vi "Export Simplified Image.vi"(11 "Control Ref Queue":T2) -> ()   [LabVIEW 2020, in "XY Plot Matrix.lvclass"]
uses:
  <vilib>/Math Plots/2D Math Plots/XY Plot Matrix/XY Plot Matrix/XY Plot Matrix.lvclass
  <vilib>/Math Plots/2D Math Plots/2D Plot/Action String/XYPlotMatrix Ctrl Act Queue.ctl
  <vilib>/Math Plots/2D Math Plots/2D Plot/Action String/XYPlotMatrix Ctrl Act Cluster.ctl
  <vilib>/Math Plots/2D Math Plots/2D Plot/Action String/2DMathPlot State Class.ctl
panel:
  in  "Warning Message":string="File path is invalid."
  in  "Save":string="Save"
  in  "Export":string="Export"
  in  "Tab Control":enum32{"Appearance", "Input & Output"}(tab)
  in  "To Clipboard":bool=TRUE
  in  "To File":bool
  in  "Help":bool
  in  "Cancel":bool
  in  "OK":bool
  in  "Hide Grid":bool
  in  "Path":path
  in  "File Format":T1(radio)
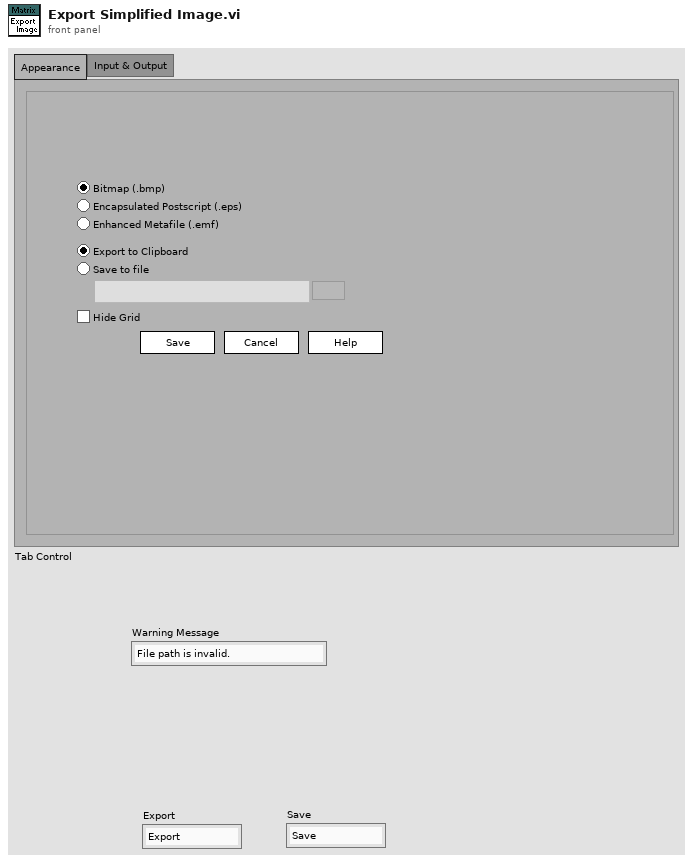
[diagram p1: front panel]
types:
  T1 = enum32{"Bitmap", "Postscript", "Metafile", "Mac PICT (.pict)"}
  T2 = typedef "XYPlotMatrix Ctrl Act Queue.ctl" = refnum<queue>
  T3 = enum8{"Enabled", "Disabled", "Disabled and Grayed Out"}
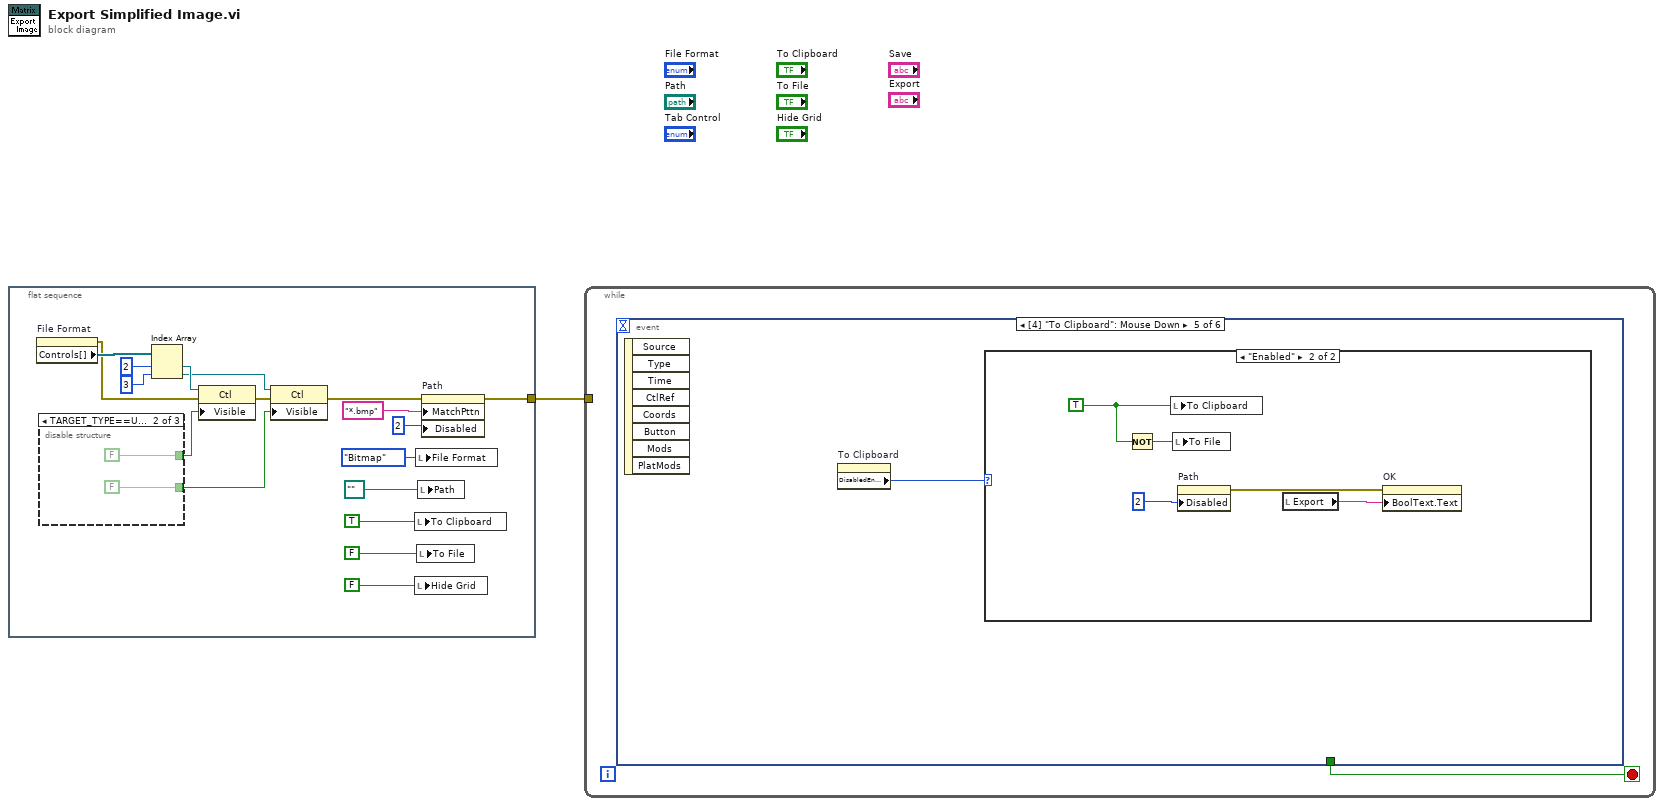
[diagram p0: block diagram]
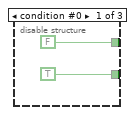
[diagram p2: hidden frame]
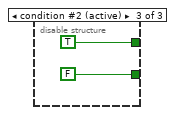
[diagram p3: hidden frame]
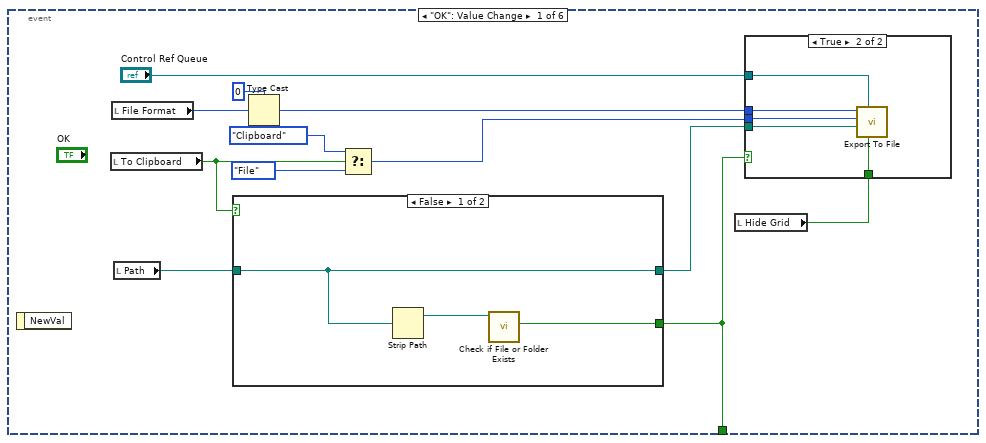
[diagram p4: hidden frame]
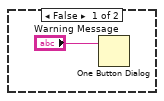
[diagram p5: hidden frame]
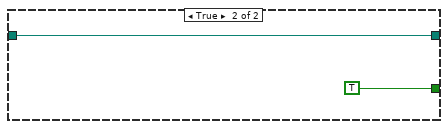
[diagram p6: hidden frame]
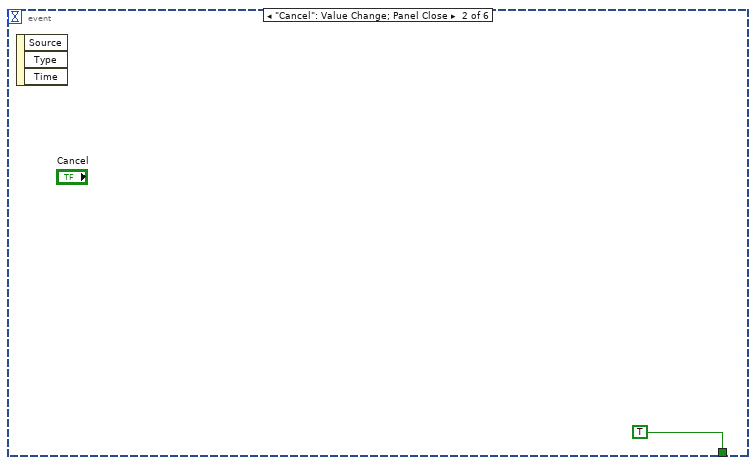
[diagram p7: hidden frame]
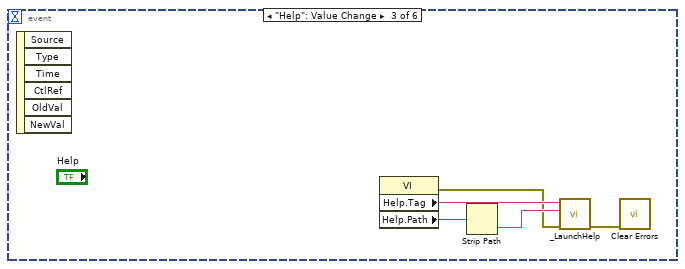
[diagram p8: hidden frame]
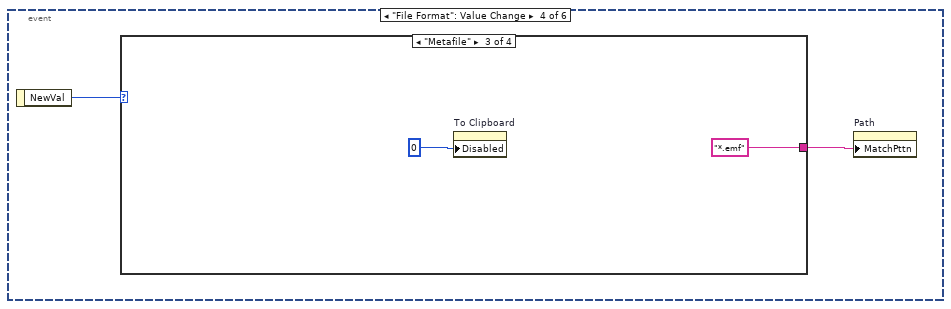
[diagram p9: hidden frame]
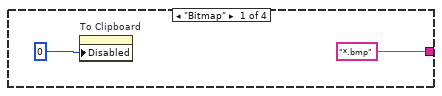
[diagram p10: hidden frame]
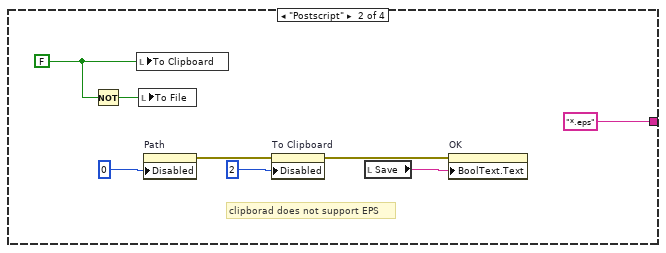
[diagram p11: hidden frame]
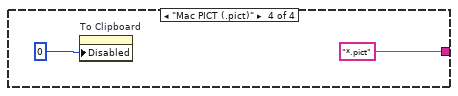
[diagram p12: hidden frame]
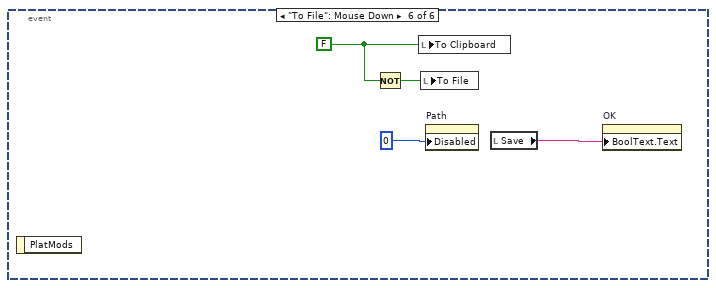
[diagram p14: hidden frame]
diagram:
  n1 = flat-sequence {
    tunnel: [w15] -> w1
    frame #0 {
      n2 = property on="File Format" class="RadioBtnsControl (strict)"() -> (error out=w7:errorcluster, "Controls[]"=w12:refnum<vi>[])  [unwired: 2 in, 1 out]
      n3 = disable-structure shown="TARGET_TYPE==Unix" {
        disable-tunnel: [FALSE ("Visible") FALSE ("Visible") TRUE ("Visible")] -> w4
        disable-tunnel: [TRUE ("Visible") FALSE ("Visible") FALSE ("Visible")] -> w3
        frame condition #0 {
        }
        frame condition #1 {
        }
        frame condition #2 (active) {
        }
      }
      n4 = Index Array(array=w12, index #1=2 ("y"), index #2=3 ("y")) -> (element #1=w11:refnum<vi>, element #2=w10:refnum<vi>)
      n5 = property class="Ctl"(reference=w11, error in=w7, "Visible"=w4) -> (error out=w9:errorcluster)  [unwired: 1 out]
      n6 = property class="Ctl"(reference=w10, error in=w9, "Visible"=w3) -> (error out=w8:errorcluster)  [unwired: 1 out]
      n7 = local write "To Clipboard"(TRUE ("To Clipboard")) -> ()
      n8 = local write "Hide Grid"(FALSE ("Hide Grid")) -> ()
      n9 = local write "File Format"(T1."Bitmap" ("File Format")) -> ()
      n10 = local write "To File"(FALSE ("To File")) -> ()
      n11 = local write "Path"(path "" ("Path")) -> ()
      n12 = property on="Path" class="Path"(error in=w8, "MatchPttn"="*.bmp" ("Browse Options:Match Pattern"), "Disabled"=u8 2) -> (error out=w15:errorcluster)  [unwired: 1 in, 1 out]
    }
  }
  n13 = while {
    tunnel: w1 -> [_]
    stop <- w26 stop-if-true
    n14 = event shown="[4] \"To Clipboard\": Mouse Down" {
      selector: _ -> [_ _ _ _ _ _]
      dyn-events: _ -> [_ _ _ _ _ _]
      timeout: _ -> [_ _ _ _ _ _]
      tunnel: [w28 TRUE _ _ _ _] -> w26
      event "OK": Value Change {
        n15 = event-data() -> ()  [unwired: 2 out]
        n16 = local read "To Clipboard"() -> (w30:bool)
        n17 = local read "File Format"() -> (w37:T1)
        n18 = local read "Path"() -> (w29:path)
        n19 = case shown="False" w30 {
          tunnel: w29 -> [w45 w49]
          tunnel: [w45 w49] -> w27
          tunnel: [w46 TRUE ("file or folder exists?")] -> w28
          frame False {
            n20 = Strip Path(path=w45) -> (stripped path=w47:path)  [unwired: 1 out]
            n21 = call <vilib>:"Check if File or Folder Exists.vi"("path"=w47) -> ("file or folder exists?"=w46:bool)  [unwired: 1 in, 9 out]
          }
          frame True {
          }
        }
        n22 = Type Cast(type=0, x=w37) -> (*(type *) &x=w35:i32)
        n23 = Select(t=enum32{"File", "Clipboard"}."Clipboard" ("Target"), s=w30, f=enum32{"File", "Clipboard"}."File") -> (s? t:f=w33:enum32{"File", "Clipboard"})
        n24 = local read "Hide Grid"() -> (w31:bool)
        n25 = case shown="True" w28 {
          tunnel: "Control Ref Queue" -> [_ w44]
          tunnel: w35 -> [_ w43]
          tunnel: w33 -> [_ w42]
          tunnel: w31 -> [_ w41]
          tunnel: w27 -> [_ w40]
          frame False {
            n26 = One Button Dialog(message="Warning Message") -> ()  [unwired: 2 out]
          }
          frame True {
            n27 = call <vilib>:"Export To File.vi"("Hide Grid"=w41, "Control Ref Queue"=w44, "Path"=w40, "Target"=w42, "File Type"=w43) -> ()  [unwired: 2 in, 5 out]
          }
        }
      }
      event "Cancel": Value Change; Panel Close {
        n28 = event-data() -> ()  [unwired: 4 out]
      }
      event "Help": Value Change {
        n29 = event-data() -> ()  [unwired: 7 out]
        n30 = property class="VI"() -> (error out=w52:errorcluster, "Help.Tag"=w54:string, "Help.Path"=w55:path)  [unwired: 2 in, 1 out]
        n31 = Strip Path(path=w55) -> (name=w53:string)  [unwired: 1 out]
        n32 = call <helpdir>:"_LaunchHelp.vi"("error in (no error)"=w52, "CHM or HLP filename (lvdialog.chm)"=w53, "HTML filename"=w54) -> ("error out"=w51:errorcluster)  [unwired: 4 out]
        n33 = call <vilib>:"Clear Errors.vi"("error in (no error)"=w51) -> ()  [unwired: 5 in, 2 out]
      }
      event "File Format": Value Change {
        n34 = event-data() -> ("NewVal"=w57:T1)  [unwired: 1 out]
        n35 = case shown="\"Metafile\"" w57 {
          tunnel: ["*.bmp" ("Browse Options:Match Pattern") "*.eps" ("Browse Options:Match Pattern") "*.emf" ("Browse Options:Match Pattern") "*.pict" ("Browse Options:Match Pattern")] -> w56
          frame "Bitmap" {
            n36 = property on="To Clipboard" class="Bool (strict)"("Disabled"=u8 0) -> ()  [unwired: 2 in, 2 out]
          }
          frame "Postscript" {
            w66 = FALSE
            # "clipborad does not support EPS"
            n37 = Not(x=w66) -> (.not. x?=w67:bool)
            n38 = local write "To Clipboard"(w66) -> ()
            n39 = local write "To File"(w67) -> ()
            n40 = property on="Path" class="Path"("Disabled"=u8 0) -> (error out=w62:errorcluster)  [unwired: 2 in, 1 out]
            n41 = property on="To Clipboard" class="Bool (strict)"(error in=w62, "Disabled"=u8 2) -> (error out=w61:errorcluster)  [unwired: 1 in, 1 out]
            n42 = local read "Save"() -> (w64:string)
            n43 = property on="OK" class="Bool"(error in=w61, "BoolText.Text"=w64) -> ()  [unwired: 1 in, 2 out]
          }
          frame "Metafile" {
            n44 = property on="To Clipboard" class="Bool (strict)"("Disabled"=u8 0) -> ()  [unwired: 2 in, 2 out]
          }
          frame "Mac PICT (.pict)" {
            n45 = property on="To Clipboard" class="Bool (strict)"("Disabled"=u8 0) -> ()  [unwired: 2 in, 2 out]
          }
        }
        n46 = property on="Path" class="Path"("MatchPttn"=w56) -> ()  [unwired: 2 in, 2 out]
      }
      event "To Clipboard": Mouse Down {
        n47 = event-data() -> ()  [unwired: 9 out]
        n48 = property on="To Clipboard" class="Bool (strict)"() -> ("DisabledEnum"=w72:T3)  [unwired: 2 in, 2 out]
        n49 = case shown="\"Enabled\"" w72 {
          frame Default {
          }
          frame "Enabled" {
            w76 = TRUE
            n50 = Not(x=w76) -> (.not. x?=w77:bool)
            n51 = local write "To Clipboard"(w76) -> ()
            n52 = local write "To File"(w77) -> ()
            n53 = property on="Path" class="Path"("Disabled"=u8 2) -> (error out=w73:errorcluster)  [unwired: 2 in, 1 out]
            n54 = local read "Export"() -> (w74:string)
            n55 = property on="OK" class="Bool"(error in=w73, "BoolText.Text"=w74) -> ()  [unwired: 1 in, 2 out]
          }
        }
      }
      event "To File": Mouse Down {
        w80 = FALSE
        n56 = event-data() -> ()  [unwired: 2 out]
        n57 = Not(x=w80) -> (.not. x?=w81:bool)
        n58 = local write "To Clipboard"(w80) -> ()
        n59 = local write "To File"(w81) -> ()
        n60 = property on="Path" class="Path"("Disabled"=u8 0) -> ()  [unwired: 2 in, 2 out]
        n61 = local read "Save"() -> (w78:string)
        n62 = property on="OK" class="Bool"("BoolText.Text"=w78) -> ()  [unwired: 2 in, 2 out]
      }
    }
  }
